vi "esp8266.vi"() -> ()   [LabVIEW 2021]
panel:
  out "remaining string":string
  out "output 1":dbl
  out "output 2":dbl
  in  "Keep Previous Location":bool
  in  "stop 2":bool
  out "2D Picture":picture
  out "data out":string
  in  "Re":bool
  out "bytes written":i32
  out "String that is sent":string
  in  "Send value 2":dbl
  in  "Send Button":bool
  in  "stop":bool
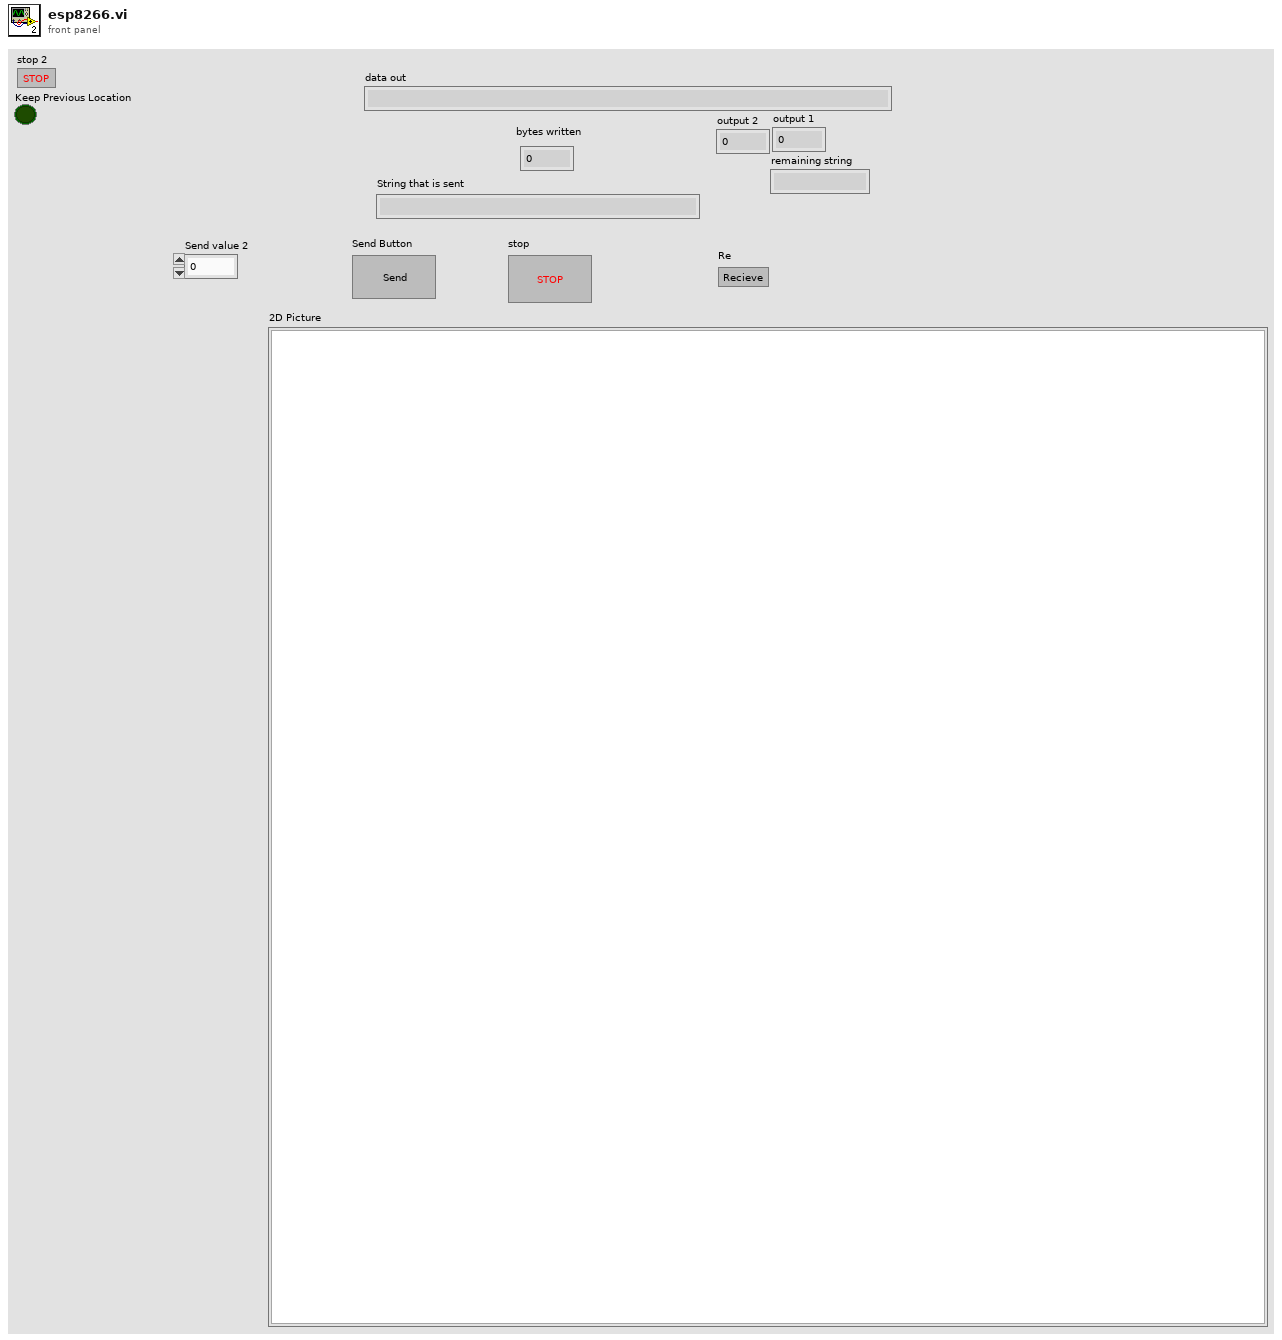
[diagram p1: front panel]
types:
  T1 = enum16{"Standard", "Buffered", "CRLF", "Immediate"}
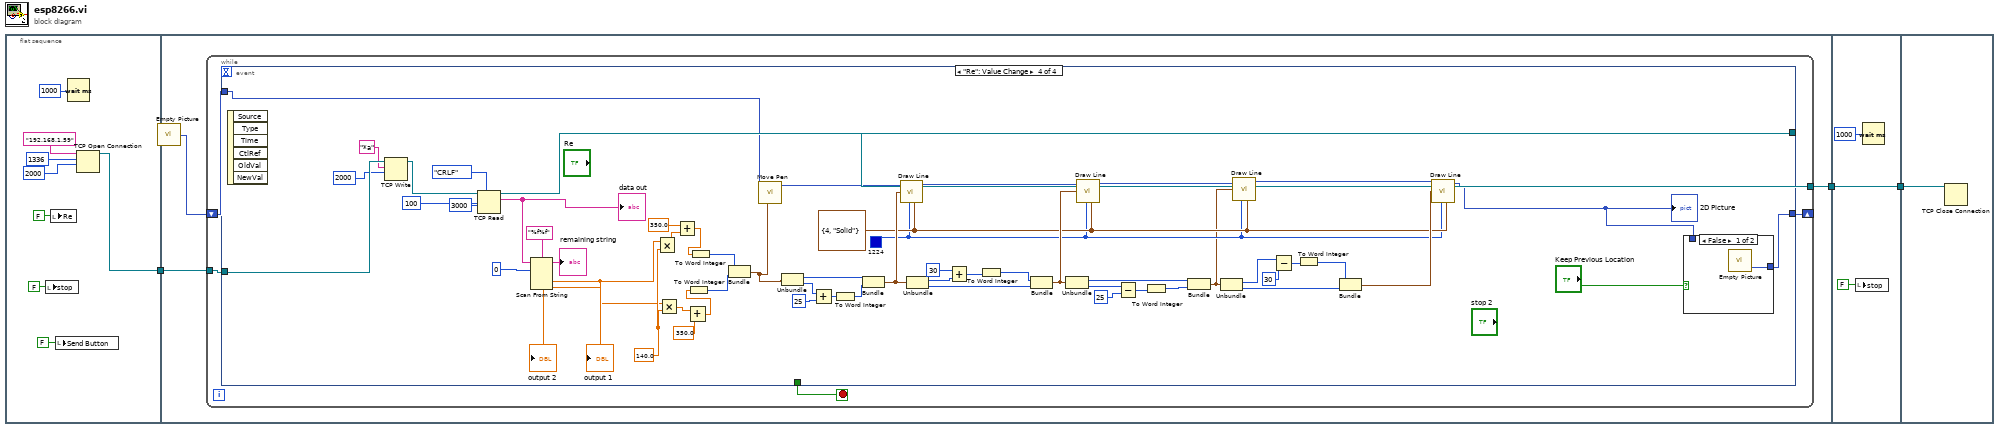
[diagram p0: block diagram]
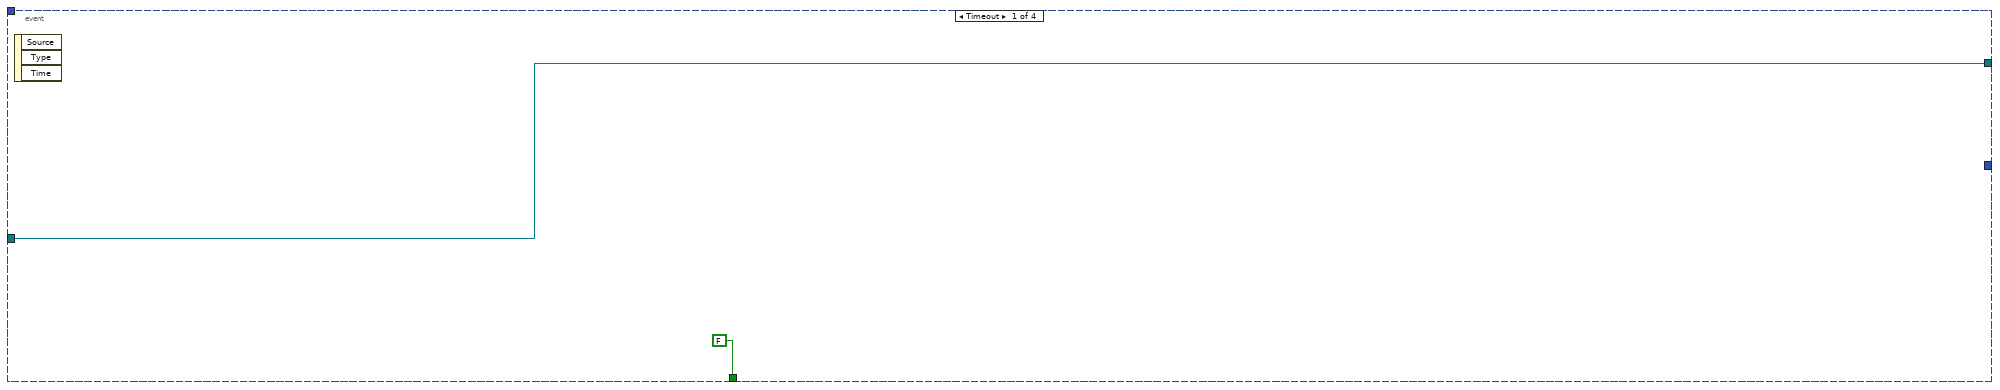
[diagram p2: hidden frame]
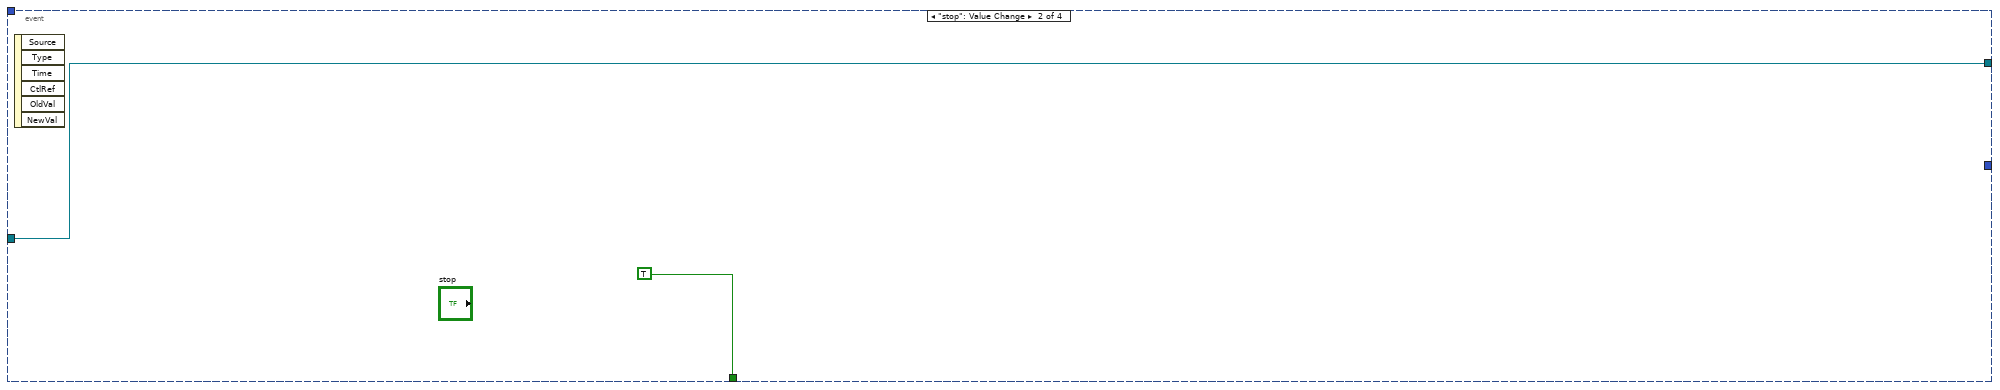
[diagram p3: hidden frame]
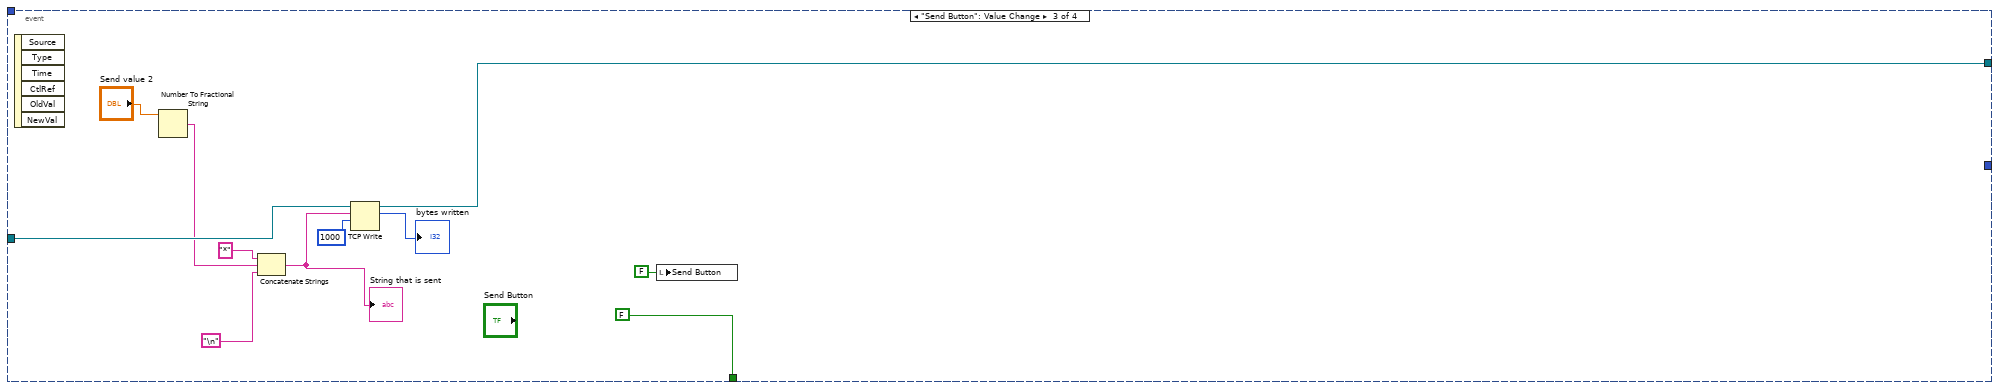
[diagram p4: hidden frame]
diagram:
  n1 = flat-sequence {
    tunnel: [w7] -> w1
    tunnel: [w14] -> w2
    tunnel: w1 -> [w13]
    tunnel: [w97] -> w3
    tunnel: w2 -> [w97]
    tunnel: w3 -> [w98]
    frame #0 {
      n2 = local write "stop"(FALSE ("stop")) -> ()
      n3 = local write "Re"(FALSE ("Re")) -> ()
      n4 = local write "Send Button"(FALSE ("Send Button")) -> ()
      n5 = Wait (ms)(milliseconds to wait=u32 1000) -> ()  [unwired: 1 out]
      n6 = TCP Open Connection(address="192.168.1.59", remote port or service name=u16 1336, timeout ms (60000)=2000) -> (connection ID=w7:refnum<k5>)  [unwired: 2 in, 1 out]
    }
    frame #1 {
      n7 = call "Empty Picture"() -> ("empty picture"=w12:picture)
      n8 = while {
        tunnel: [w18] -> w14
        tunnel: w13 -> [w17]
        shift-right: [w15] -> _
        shift-left: w12 -> [w16]
        stop <- w19 stop-if-true
        n9 = event shown="[3] \"Re\": Value Change" {
          selector: _ -> [_ _ _ _]
          dyn-events: _ -> [_ _ _ _]
          timeout: _ -> [_ _ _ _]
          tunnel: [FALSE TRUE FALSE _] -> w19
          tunnel: [w20 w23 w26 w86] -> w18
          tunnel: w17 -> [w20 w23 w32 w92]
          tunnel: w16 -> [_ _ _ w46]
          tunnel: [_ _ _ w45] -> w15
          event Timeout {
            n10 = event-data() -> ()  [unwired: 1 in, 3 out]
          }
          event "stop": Value Change {
            n11 = event-data() -> ()  [unwired: 1 in, 6 out]
          }
          event "Send Button": Value Change {
            n12 = event-data() -> ()  [unwired: 1 in, 6 out]
            n13 = Number To Fractional String(number="Send value 2") -> (F-format string=w27:string)  [unwired: 3 in]
            n14 = Concatenate Strings("*" ("string"), w27, "\n") -> (w29:string)
            "String that is sent" <- w29
            n15 = TCP Write(connection ID=w32, data in=w29, 9:1000 ("timeout ms (25000)")) -> (connection ID out=w26:refnum<k5>, bytes written=→"bytes written":i32)  [unwired: 1 in, 1 out]
            n16 = local write "Send Button"(FALSE ("Send Button")) -> ()
          }
          event "Re": Value Change {
            w48 = 140.0 ("y")
            w57 = u32 1224 ("color(black)")
            w58 = cluster{i32, enum16{"Solid"}} {4, enum."Solid"}
            n17 = event-data() -> ()  [unwired: 1 in, 6 out]
            n18 = TCP Write(connection ID=w92, data in="*a", 9:2000 ("timeout ms (25000)")) -> (connection ID out=w89:refnum<k5>)  [unwired: 1 in, 2 out]
            n19 = TCP Read(connection ID=w89, bytes to read=100, 7:T1."CRLF" ("mode (standard)"), 9:3000 ("timeout ms (25000)")) -> (connection ID out=w86:refnum<k5>, data out=w42:string)  [unwired: 1 in, 1 out]
            "data out" <- w42
            n20 = Scan From String "Scan From String"(format string="%f%f", input string=w42, initial scan location=u32 0) -> (remaining string=→"remaining string":string, output 1=w47:dbl, output 2=w43:dbl)  [unwired: 3 in, 2 out]
            "output 2" <- w43
            "output 1" <- w47
            n21 = Multiply(x=w47, y=w48) -> (x*y=w40:dbl)
            n22 = Multiply(x=w43, y=w48) -> (x*y=w37:dbl)
            n23 = Add(x=350.0, y=w40) -> (x+y=w39:dbl)
            n24 = Add(x=w37, y=350.0) -> (x+y=w38:dbl)
            n25 = To Word Integer(number=w38) -> (16bit integer=w82:i16)
            n26 = To Word Integer(number=w39) -> (16bit integer=w83:i16)
            n27 = Bundle(w83, w82) -> (w56:cluster{i16, i16})  [unwired: 1 in]
            n28 = call <vilib>:"Move Pen.vi"("new position"=w56, "picture"=w46) -> ("new picture"=w54:picture)  [unwired: 3 in]
            n29 = Unbundle(w56) -> (w78:i16, w77:i16)
            n30 = Add(x=w77, y=i16 25) -> (x+y=w81:i16)
            n31 = To Word Integer(number=w81) -> (16bit integer=w79:i16)
            n32 = Bundle(w78, w79) -> (w76:cluster{i16, i16})  [unwired: 1 in]
            n33 = call <vilib>:"Draw Line.vi"("picture"=w54, "end point"=w76, "color(black)"=w57, "pen"=w58) -> ("new picture"=w53:picture)  [unwired: 5 in]
            n34 = Unbundle(w76) -> (w74:i16, w72:i16)
            n35 = Add(x=i16 30, y=w74) -> (x+y=w75:i16)
            n36 = To Word Integer(number=w75) -> (16bit integer=w71:i16)
            n37 = Bundle(w71, w72) -> (w70:cluster{i16, i16})  [unwired: 1 in]
            n38 = Unbundle(w70) -> (w65:i16, w69:i16)
            n39 = call <vilib>:"Draw Line.vi"("picture"=w53, "end point"=w70, "color(black)"=w57, "pen"=w58) -> ("new picture"=w52:picture)  [unwired: 5 in]
            n40 = Subtract(x=w69, y=i16 25) -> (x-y=w67:i16)
            n41 = To Word Integer(number=w67) -> (16bit integer=w66:i16)
            n42 = Bundle(w65, w66) -> (w49:cluster{i16, i16})  [unwired: 1 in]
            n43 = Unbundle(w49) -> (w64:i16, w60:i16)
            n44 = call <vilib>:"Draw Line.vi"("picture"=w52, "end point"=w49, "color(black)"=w57, "pen"=w58) -> ("new picture"=w51:picture)  [unwired: 5 in]
            n45 = Subtract(x=w64, y=i16 30) -> (x-y=w62:i16)
            n46 = To Word Integer(number=w62) -> (16bit integer=w61:i16)
            n47 = Bundle(w61, w60) -> (w59:cluster{i16, i16})  [unwired: 1 in]
            n48 = call <vilib>:"Draw Line.vi"("picture"=w51, "end point"=w59, "color(black)"=w57, "pen"=w58) -> ("new picture"=w50:picture)  [unwired: 5 in]
            "2D Picture" <- w50
            n49 = case shown="False" "Keep Previous Location" {
              tunnel: [w93 w94] -> w45
              tunnel: w50 -> [_ w94]
              frame False {
                n50 = call "Empty Picture"() -> ("empty picture"=w93:picture)
              }
              frame True {
              }
            }
          }
        }
      }
    }
    frame #2 {
      n51 = local write "stop"(FALSE ("stop")) -> ()
      n52 = Wait (ms)(milliseconds to wait=u32 1000) -> ()  [unwired: 1 out]
    }
    frame #3 {
      n53 = TCP Close Connection(connection ID=w98) -> ()  [unwired: 2 in, 2 out]
    }
  }
